vi "Master.vi"() -> ()   [LabVIEW 2020]
uses:
  <vilib>/Platform/TimedLoop/XDataNode/timing_clust.ctl
  <vilib>/Platform/TimedLoop/XDataNode/nitl_modes.ctl
  <vilib>/Platform/TimedLoop/XDataNode/wakeup.ctl
  37583fcc-cec8-480d-a6d0-1da09da3d0dd.vi
  <vilib>/Instr/_visa.llb/VISA Configure Serial Port (Instr).vi
  <vilib>/platform/TimedLoop/XDataNode/XDataNode.xnode
  <vilib>/Platform/TimedLoop/XDataNode/XDNodeRunTimeDep.lvlib
panel:
  in  "Start":bool
  in  "VISA resource name":refnum<visa-resource-name>
  out "Send String":string
  out "Error Out":errorcluster
  out "Distance":dbl
  out "Move Time":u32
  in  "Pixels":cluster{"x":dbl, "y":dbl}[](array[cluster])
  out "Progress":dbl(slide) scale=0.0..1.0
  out "Current XY":cluster{"X":dbl, "Y":dbl}
  out "XY Graph":cluster{dbl[], dbl[]}[](graph)
  in  "Stop":bool
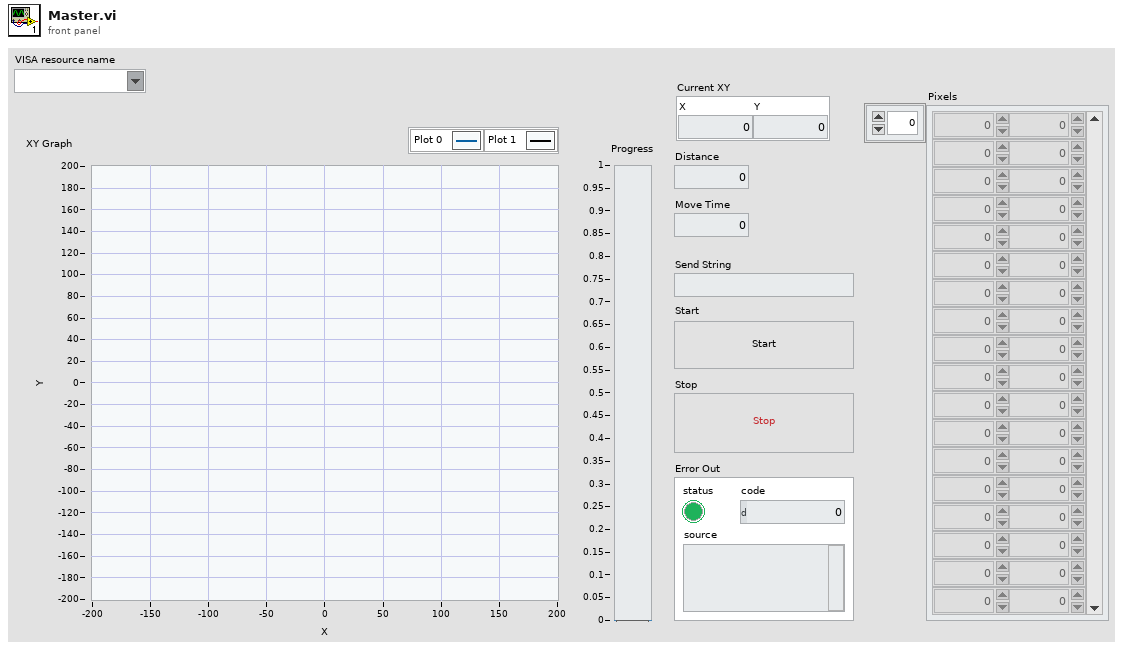
[diagram p1: front panel]
types:
  T1 = typedef "XDNodeRunTimeDep.lvlib/timing_clust.ctl" = cluster{"Expected End [f-1]":u64, "Actual End [f-1]":u64, "Finished Late? [f-1]":bool, "Expected End [i-1]":u64, "Actual End [i-1]":u64, "Finished Late? [i-1]":bool, "Expected Start [i]":u64, "Actual Start [i]":u64, "Expected Start [f]":u64, "Actual Start [f]":u64, "Source Name":string, "Structure Name":string, "Period":i64, "Deadline":i64, "Offset":i64, "Start":i64, "Priority":i32, "Timeout":i32, "Mode":T2, "Wakeup Reason":T3, "Error":errorcluster, "Source Type":string, "Secondary Source Type":string, "Global End Time":u64, "Global Start Time":u64, "Frame Duration":u64, "Iteration Duration":u64, "Assigned CPU":i32, "I/O Scan Engine Mode":u32}
  T2 = typedef "XDNodeRunTimeDep.lvlib/nitl_modes.ctl" = enum32{"No Change", "Process missed periods, maintain original phase", "Discard missed periods, maintain original phase", "Process missed periods, ignore original phase", "Discard missed periods, ignore original phase"}
  T3 = typedef "XDNodeRunTimeDep.lvlib/wakeup.ctl" = enum32{"Normal", "Aborted", "Asynchronous wakeup", "Timing source error", "Timed loop error", "Timeout"}
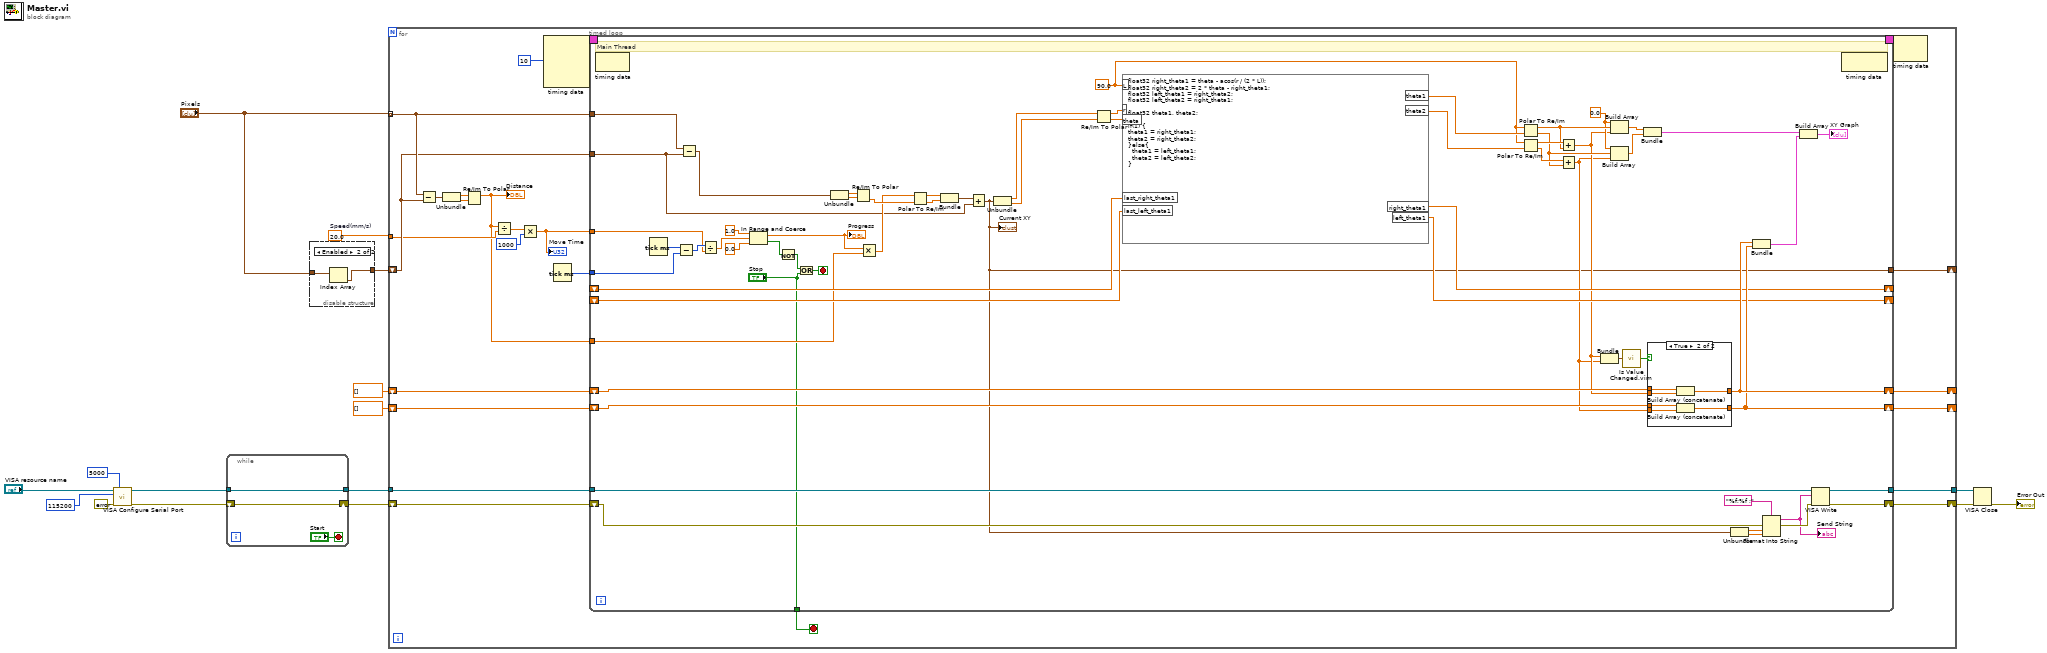
[diagram p0: block diagram]
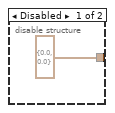
[diagram p2: hidden frame]
diagram:
  w15 = 20.0  # Speed(mm/s)
  n1 = call-poly "VISA Configure Serial Port"("VISA resource name"="VISA resource name", "timeout (10sec)"=u32 5000, "baud rate (9600)"=u32 115200, "error in (no error)"=errorcluster {"status"=FALSE, "code"=0, "source"=""}) -> ("VISA resource name out"=w2:refnum<visa-resource-name>, "error out"=w5:errorcluster)  [unwired: 10 in]
  n2 = while {
    shift-right: [w19] -> w4
    shift-left: w5 -> [w19]
    tunnel: [w18] -> w3
    tunnel: w2 -> [w18]
    stop <- "Start" stop-if-true
  }
  n3 = disable-structure shown="Enabled" {
    disable-tunnel: [cluster{dbl, dbl} {0.0, 0.0} w21] -> w16
    disable-tunnel: "Pixels" -> [_ w22]
    frame Disabled {
    }
    frame Enabled {
      n4 = Index Array(array=w22) -> (element=w21:cluster{"x":dbl, "y":dbl})  [unwired: 1 in]
    }
  }
  n5 = for {
    tunnel: "Pixels" -> [w37] mode=indexing
    shift-right: [w43] -> _
    shift-left: w16 -> [w36]
    tunnel: w15 -> [w35]
    shift-right: [w30] -> _
    shift-left: dbl[] [] -> [w31]
    shift-right: [w29] -> _
    shift-left: dbl[] [] -> [w28]
    shift-right: [w25] -> w9
    shift-left: w4 -> [w27]
    tunnel: w3 -> [w26]
    tunnel: [w24] -> w8
    stop <- w23 stop-if-true
    n6 = Subtract(x=w37, y=w36) -> (x-y=w40:cluster{"x":dbl, "y":dbl})
    n7 = Unbundle(w40) -> ("x"=w39:dbl, "y"=w38:dbl)
    n8 = Re/Im To Polar(2:w38, 3:w39) -> (1:w33:dbl)  [unwired: 1 out]
    "Distance" <- w33
    n9 = Divide(x=w33, y=w35) -> (x/y=w41:dbl)
    n10 = Multiply(x=w41, y=u32 1000 ("millisecond timer value")) -> (x*y=w34:dbl)
    "Move Time" <- w34
    n11 = node-c288(i64 10 ("Period")) -> (w46:T1)  [unwired: 3 in]
    n12 = Tick Count (ms)() -> (millisecond timer value=w32:u32)
    n13 = timed-loop {
      timing: w46 -> [_]
      timing-out: [_] -> w45
      shift-right: [w80] -> w30
      shift-left: w31 -> [w85]
      shift-right: [w79] -> w29
      shift-left: w28 -> [w84]
      shift-right: [w70] -> _
      shift-left: _ -> [w69]
      shift-right: [w71] -> _
      shift-left: _ -> [w68]
      tunnel: w37 -> [w66]
      tunnel: [w49] -> w43
      tunnel: w36 -> [w65]
      tunnel: w34 -> [w64]
      tunnel: w33 -> [w63]
      tunnel: w32 -> [w62]
      shift-right: [w56] -> w25
      shift-left: w27 -> [w58]
      tunnel: w26 -> [w57]
      tunnel: [w55] -> w24
      tunnel: ["Stop"] -> w23
      stop <- w51 stop-if-true
      w89 = 0.0 ("element")
      w86 = 90.0 ("input variable")
      # "Main Thread"
      n14 = node-c288() -> ()  [unwired: 1 in, 1 out]
      n15 = Tick Count (ms)() -> (millisecond timer value=w108:u32)
      n16 = Subtract(x=w108, y=w62) -> (x-y=w76:u32)
      n17 = Subtract(x=w66, y=w65) -> (x-y=w107:cluster{"x":dbl, "y":dbl})
      n18 = Divide(x=w76, y=w64) -> (x/y=w75:dbl)
      n19 = In Range and Coerce(upper limit=1.0 ("lower limit"), x=w75, lower limit=0.0) -> (coerced(x)=w72:dbl, In Range?=w67:bool)
      "Progress" <- w72
      n20 = Not(x=w67) -> (.not. x?=w52:bool)
      n21 = Or(x=w52, y="Stop") -> (x .or. y?=w51:bool)
      n22 = Unbundle(w107) -> ("x"=w106:dbl, "y"=w105:dbl)
      n23 = Re/Im To Polar(2:w105, 3:w106) -> (0:w104:dbl)  [unwired: 1 out]
      n24 = Multiply(x=w72, y=w63) -> (x*y=w97:dbl)
      n25 = Polar To Re/Im(2:w104, 3:w97) -> (0:w102:dbl, 1:w103:dbl)
      n26 = Bundle(w103, w102) -> (w101:cluster{dbl, dbl})  [unwired: 1 in]
      n27 = Add(x=w101, y=w65) -> (x+y=w49:cluster{dbl, dbl})
      "Current XY" <- w49
      n28 = Unbundle(w49) -> (w100:dbl, w99:dbl)
      n29 = Re/Im To Polar(2:w99, 3:w100) -> (0:w98:dbl, 1:w96:dbl)
      n30 = formula code="float32 right_theta1 = theta - acos(r / (2 * L));\nfloat32 right_theta2 = 2 * theta - right_theta1;\nfloat32 left_theta1 = right_theta2;\nfloat32 left_theta2 = right_theta1;\n\nfloat32 theta1, theta2;\n\nif(1) {\ntheta1 = right_theta1;\ntheta2 = right_theta2;\n}else{\n  theta1 = left_theta1;\n  theta2 = left_theta2;\n}"("r"=w96, "theta"=w98, "L"=w86, "last_right_theta1"=w69, "last_left_theta1"=w68) -> ("theta1"=w88:sgl, "theta2"=w87:sgl, "right_theta1"=w70:sgl, "left_theta1"=w71:sgl)
      n31 = Polar To Re/Im(2:w88, 3:w86) -> (0:w92:dbl, 1:w93:dbl)
      n32 = Polar To Re/Im(2:w87, 3:w86) -> (0:w94:dbl, 1:w95:dbl)
      n33 = Add(x=w95, y=w93) -> (x+y=w54:dbl)
      n34 = Add(x=w94, y=w92) -> (x+y=w53:dbl)
      n35 = Bundle(w54, w53) -> (w83:cluster{dbl, dbl})  [unwired: 1 in]
      n36 = Build Array(w89, w93, w54) -> (w91:dbl[])
      n37 = Build Array(w89, w92, w53) -> (w90:dbl[])
      n38 = call "Is Value Changed.vim"("value"=w83) -> ("changed or first call?"=w82:bool)
      n39 = Bundle(w91, w90) -> (w81:cluster{dbl[], dbl[]})  [unwired: 1 in]
      n40 = case shown="True" w82 {
        tunnel: w54 -> [_ w116]
        tunnel: w53 -> [_ w115]
        tunnel: [w110 w114] -> w80
        tunnel: [w109 w113] -> w79
        tunnel: w85 -> [w110 w112]
        tunnel: w84 -> [w109 w111]
        frame False {
        }
        frame True {
          n41 = Build Array (concatenate)(w112, w116) -> (w114:dbl[])
          n42 = Build Array (concatenate)(w111, w115) -> (w113:dbl[])
        }
      }
      n43 = Unbundle(w49) -> (w48:dbl, w47:dbl)
      n44 = Bundle(w80, w79) -> (w78:cluster{dbl[], dbl[]})  [unwired: 1 in]
      n45 = Format Into String(format string="%f;%f ;", error in=w58, w48, w47) -> (resulting string=w59:string, error out=w60:errorcluster)  [unwired: 1 in]
      "Send String" <- w59
      n46 = Build Array(w81, w78) -> (→"XY Graph":cluster{dbl[], dbl[]}[])
      n47 = VISA Write(VISA resource name=w57, write buffer=w59, error in (no error)=w60) -> (VISA resource name out=w55:refnum<visa-resource-name>, error out=w56:errorcluster)  [unwired: 1 out]
      n48 = node-c288() -> ()  [unwired: 1 in, 1 out]
    }
    n49 = node-c288(w45) -> ()  [unwired: 1 out]
  }
  n50 = VISA Close(VISA resource name=w8, error in (no error)=w9) -> (error out=→"Error Out":errorcluster)
